vi "id.From JSON Tree.vi"(8 "error in (no error)":errorcluster, 10 "JSON Value in":refnum<class "JSON Value.lvclass">, 11 "id in":refnum<class "id.lvclass">) -> (0 "error out":errorcluster, 3 "id out":refnum<class "id.lvclass">)   [LabVIEW 2016, in "id.lvclass"]
uses:
  id.lvclass
  <vilib>/NI/JSON Support for LabVIEW/JSON Value/JSON Value.lvclass
  id.lvclass/id.ctl
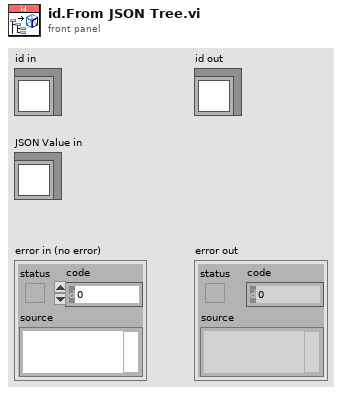
[diagram p1: front panel]
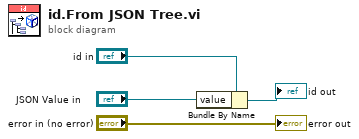
[diagram p0: block diagram]
diagram:
  n1 = Bundle By Name(cluster="id in", "value"="JSON Value in") -> (→"id out":refnum<class "id.lvclass">)
  "error out" <- "error in (no error)"
